vi "cut.vi"(3 "start/duration format":u16(ring)=1 items=["Samples", "Relative Time"], 4 "data info template":refnum<vi>, 5 "input":waveform(dbl), 6 "open interval? (T)":bool, 7 "cut  end":dbl=0.001 format="%#.6e", 8 "Begin offset":dbl=0.01 format="%#.6e") -> (0 "Part of input":waveform(dbl), 1 "short cut data lables":string, 2 "cut data lables":string)   [LabVIEW 2014]
uses:
  <vilib>/Waveform/WDTOps.llb/WDT Get Waveform Subset DBL.vi
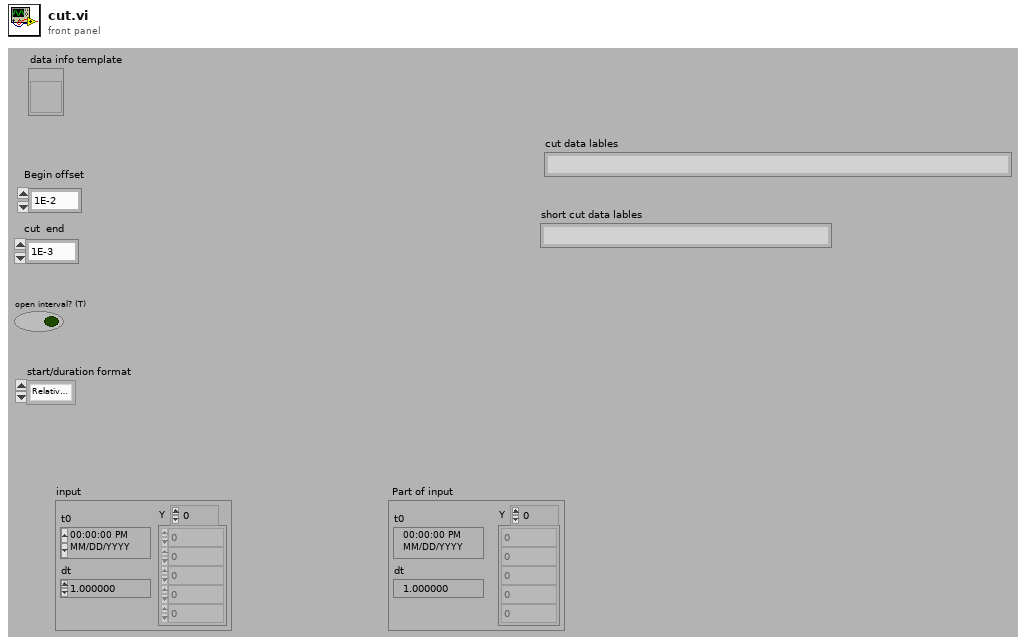
[diagram p1: front panel]
types:
  T1 = cluster{"data path":string, "ADCintercadr_s":dbl, "data info":cluster{"use or not *.info.txt?":i16, "probe name":string, "signal type":string, "Unit":string, "variable":string, "attenuation factor":dbl, "amplification factor":dbl, "extracoef#1":dbl, "extracoef#2":dbl, "U cascade, kV":string, "probe area, cm2":dbl, "plasma, a.m.u.":dbl}, "channel_name":string, "channels_in_file":i32}
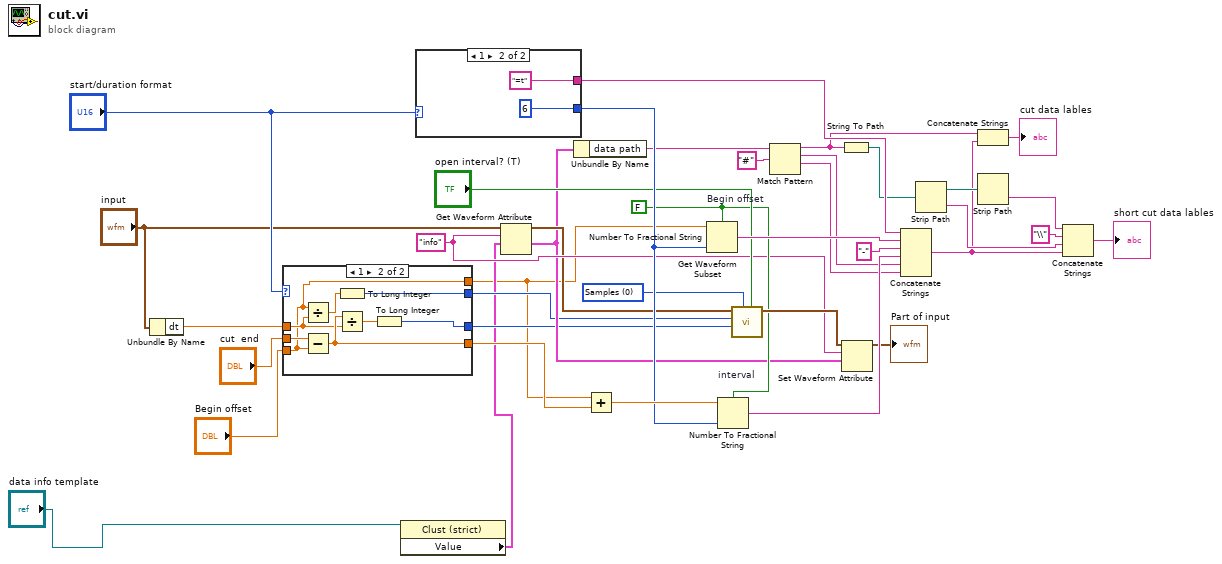
[diagram p0: block diagram]
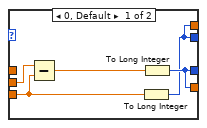
[diagram p2: hidden frame]
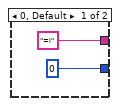
[diagram p3: hidden frame]
diagram:
  w7 = u16 0 items=["Samples", "Relative Time"] ("start/duration format")
  w18 = FALSE ("use system decimal point (T)")
  w16 = "info" ("name")
  n1 = Unbundle By Name("input") -> ("dt"=w5:dbl)
  n2 = case shown="1" "start/duration format" {
    tunnel: "cut  end" -> [w43 w51]
    tunnel: [w41 w45] -> w11
    tunnel: "Begin offset" -> [w40 w44]
    tunnel: [w39 w47] -> w9
    tunnel: w5 -> [_ w49]
    tunnel: [w41 w50] -> w4
    tunnel: [w39 w44] -> w1
    frame 0, Default {
      n3 = Subtract(x=w43, y=w40) -> (x-y=w42:dbl)
      n4 = To Long Integer(number=w40) -> (32bit integer=w39:i32)
      n5 = To Long Integer(number=w42) -> (32bit integer=w41:i32)
    }
    frame 1 {
      n6 = Divide(x=w44, y=w49) -> (x/y=w48:dbl)
      n7 = Subtract(x=w51, y=w44) -> (x-y=w50:dbl)
      n8 = To Long Integer(number=w48) -> (32bit integer=w47:i32)
      n9 = Divide(x=w50, y=w49) -> (x/y=w46:dbl)
      n10 = To Long Integer(number=w46) -> (32bit integer=w45:i32)
    }
  }
  n11 = property on="Property Node" class="Clust (strict)"(reference="data info template") -> ("Value"=w3:T1)  [unwired: 1 in, 2 out]
  n12 = case shown="1" "start/duration format" {
    tunnel: [i16 0 ("precision (6)") i16 6 ("precision (6)")] -> w34
    tunnel: ["=i" "=t"] -> w29
    frame 0, Default {
    }
    frame 1 {
    }
  }
  n13 = Get Waveform Attribute(5:w3, 6:w16, 7:"input") -> (1:w14:T1, 3:w15:waveform(dbl))  [unwired: 1 in, 2 out]
  n14 = Unbundle By Name(w14) -> ("data path"=w17:string)
  n15 = Add(x=w1, y=w4) -> (x+y=w35:dbl)
  n16 = Number To Fractional String "Begin offset"(use system decimal point (T)=w18, number=w1, precision (6)=w34) -> (F-format string=w37:string)  [unwired: 1 out]
  n17 = Number To Fractional String "interval"(use system decimal point (T)=w18, number=w35, precision (6)=w34) -> (F-format string=w38:string)  [unwired: 1 out]
  n18 = call-poly <vilib>:"Get Waveform Subset.vi"("open interval? (T)"="open interval? (T)", "start/duration format"=w7, "duration"=w11, "start samples/time"=w9, "waveform in"=w15) -> ("waveform out"=w33:waveform(dbl))  [unwired: 1 in, 3 out]
  n19 = Match Pattern(string=w17, regular expression="#") -> (before substring=w27:string, match substring=w28:string, after substring=w20:string)  [unwired: 1 in, 1 out]
  n20 = String To Path(string=w27) -> (path=w26:path)
  n21 = Set Waveform Attribute(5:w14, 6:w16, 7:w33) -> (3:→"Part of input":waveform(dbl))  [unwired: 1 in, 2 out]
  n22 = Concatenate Strings(w29, w37, "-", w38, w28, w20) -> (w19:string)
  n23 = Strip Path(path=w26) -> (stripped path=w23:path, name=w25:string)
  n24 = Concatenate Strings(w27, w19) -> (→"cut data lables":string)
  n25 = Strip Path(path=w23) -> (name=w21:string)  [unwired: 1 out]
  n26 = Concatenate Strings(w21, "\\" ("string"), w25, w19) -> (→"short cut data lables":string)
